vi "Move Selection.vi"(5 "XY Graph Ref":refnum<vi>, 8 "error in (no error)":errorcluster, 9 "Coords":T1, 11 "Xinformation In":T2) -> (0 "error out":errorcluster, 3 "Xinformation Out":T2)   [LabVIEW 2020, in "Overview XControl.xctl"]
doc: "This vi handles when the user has grabbed the timline and dragged to the left and right. This also prevents the user from dragging too far to the right or the left (outside the timeline span)"
uses:
  Overview XControl.xctl
  <vilib>/Utility/miscctls.llb/LVPoint32TypeDef.ctl
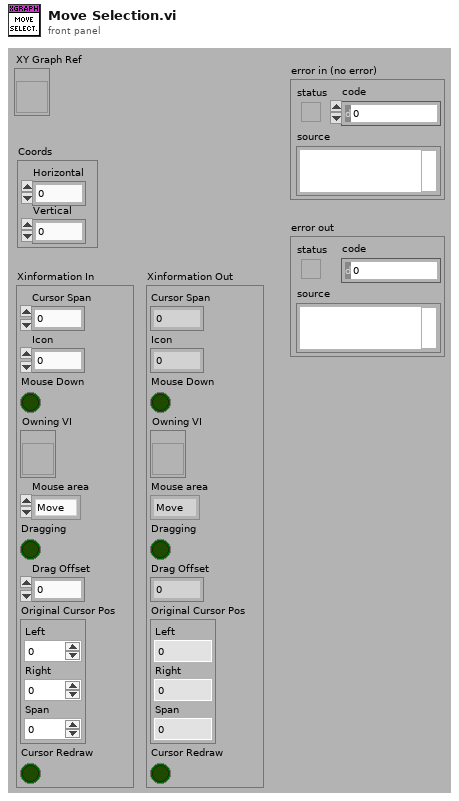
[diagram p1: front panel]
types:
  T1 = typedef "LVPoint32TypeDef.ctl" = cluster{"Horizontal":i32, "Vertical":i32}
  T2 = cluster{"Cursor Span":dbl, "Icon":u16, "Mouse Down":bool, "Owning VI":refnum<vi>, "Mouse area":enum16{"Move", "left cursor", "right cursor", "none"}, "Dragging":bool, "Drag Offset":dbl, "Original Cursor Pos":cluster{"Left":dbl, "Right":dbl, "Span":dbl}, "Cursor Redraw":bool}
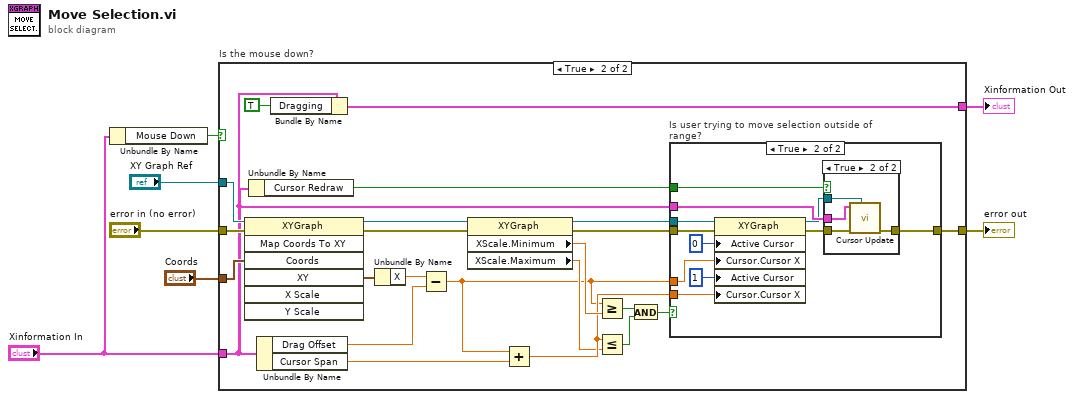
[diagram p0: block diagram]
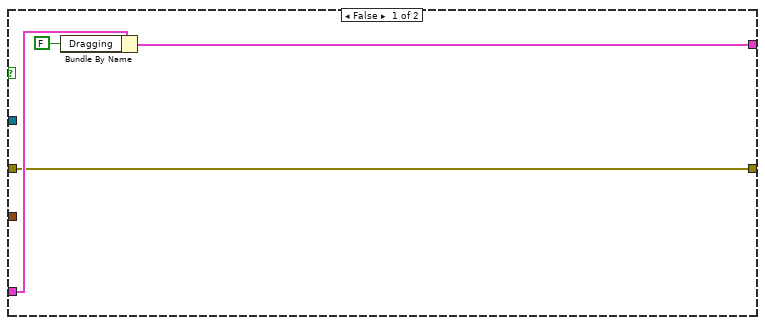
[diagram p2: hidden frame]
diagram:
  n1 = Unbundle By Name("Xinformation In") -> ("Mouse Down"=w6:bool)
  n2 = case "Is the mouse down?" shown="True" w6 {
    tunnel: "Coords" -> [_ w23]
    tunnel: "Xinformation In" -> [w10 w13]
    tunnel: [w9 w31] -> w5
    tunnel: "XY Graph Ref" -> [_ w20]
    tunnel: "error in (no error)" -> [w8 w19]
    tunnel: [w8 w16] -> w1
    frame False {
      n3 = Bundle By Name(cluster=w10, "Dragging"=FALSE) -> (w9:T2)
    }
    frame True {
      n4 = invoke on="Invoke Node" class="XYGraph" method="Map Coords To XY"(reference=w20, error in=w19, "Coords"=w23) -> (reference out=w15:refnum<vi>, error out=w18:errorcluster, "XY"=w33:cluster{"X":dbl, "Y":dbl})  [unwired: 4 in, 4 out]
      n5 = Unbundle By Name(w13) -> ("Cursor Redraw"=w12:bool)
      n6 = Unbundle By Name(w13) -> ("Drag Offset"=w32:dbl, "Cursor Span"=w34:dbl)
      n7 = Bundle By Name(cluster=w13, "Dragging"=TRUE) -> (w31:T2)
      n8 = Unbundle By Name(w33) -> ("X"=w22:dbl)
      n9 = Subtract(x=w22, y=w32) -> (x-y=w21:dbl)
      n10 = property on="Property Node" class="XYGraph"(reference=w15, error in=w18) -> (reference out=w14:refnum<vi>, error out=w17:errorcluster, "XScale.Minimum"=w29:dbl, "XScale.Maximum"=w26:dbl)
      n11 = Add(x=w21, y=w34) -> (x+y=w27:dbl)
      n12 = Greater Or Equal?(x=w21, y=w29) -> (x >= y?=w28:bool)
      n13 = Less Or Equal?(x=w27, y=w26) -> (x <= y?=w25:bool)
      n14 = And(x=w28, y=w25) -> (x .and. y?=w24:bool)
      n15 = case "Is user trying to move selection outside of range?" shown="True" w24 {
        tunnel: w27 -> [_ w45]
        tunnel: w21 -> [_ w43]
        tunnel: w13 -> [_ w42]
        tunnel: w14 -> [_ w41]
        tunnel: w17 -> [w35 w38]
        tunnel: [w35 w39] -> w16
        tunnel: w12 -> [_ w37]
        frame False {
        }
        frame True {
          n16 = property on="Property Node" class="XYGraph"(reference=w41, error in=w38, "Active Cursor"=u32 0, "Cursor.Cursor X"=w43, "Active Cursor"=u32 1, "Cursor.Cursor X"=w45) -> (reference out=w36:refnum<vi>, error out=w40:errorcluster)
          n17 = case shown="True" w37 {
            tunnel: w42 -> [_ w51]
            tunnel: w36 -> [_ w50]
            tunnel: w40 -> [w47 w49]
            tunnel: [w47 w48] -> w39
            frame False {
            }
            frame True {
              n18 = call "Cursor Update.vi"("XY Graph Ref"=w50, "error in (no error)"=w49, "Xinformation In"=w51) -> ("error out"=w48:errorcluster)  [unwired: 7 in, 1 out]
            }
          }
        }
      }
    }
  }
  "Xinformation Out" <- w5
  "error out" <- w1
